vi "Write serialProtocolFactory.vi"(10 "serialProtocolFactory":refnum<class "ISerialProtocolFactory.lvclass">, 11 "SerialCommunicator in":refnum<class "SerialCommunicator.lvclass">) -> (3 "SerialCommunicator out":refnum<class "SerialCommunicator.lvclass">)   [LabVIEW 2013, in "SerialProtocols.lvlib" / "SerialCommunicator.lvclass"]
uses:
  <userlib>/Common/SerialProtocols/SerialCommunicator/SerialCommunicator.lvclass
  <userlib>/Common/SerialProtocols/SerialProtocolFactory/ISerialProtocolFactory/ISerialProtocolFactory.lvclass
  <userlib>/Common/SerialProtocols/SerialCommunicator/SerialCommunicator.lvclass/SerialCommunicator.ctl
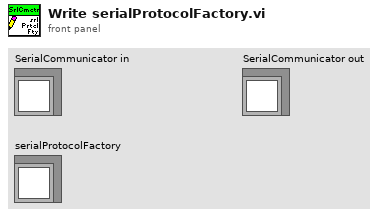
[diagram p1: front panel]
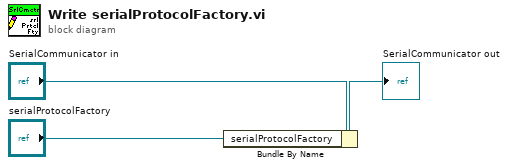
[diagram p0: block diagram]
diagram:
  n1 = Bundle By Name(cluster="SerialCommunicator in", "serialProtocolFactory"="serialProtocolFactory") -> (→"SerialCommunicator out":refnum<class "SerialCommunicator.lvclass">)
